vi "Write PWM.vi"(8 "Back Right":dbl, 9 "Front Right":dbl, 10 "Back Left":dbl, 11 "Front Left":dbl) -> ()   [LabVIEW 2017]
uses:
  <vilib>/myRIO/Instrument Drivers/Onboard IO/DIO/typedefs/DIO Reference.ctl
  <vilib>/myRIO/Common/Instrument Driver Framework/Utilities/typedefs/myRIO Generic Hardware Reference.ctl
  <vilib>/myRIO/Common/Instrument Driver Framework/Utilities/typedefs/Hardware Version Enum.ctl
  <vilib>/myRIO/Common/Instrument Driver Framework/Utilities/typedefs/myRIO v1.0 Reference.ctl
  <vilib>/myRIO/Common/Instrument Driver Framework/Utilities/typedefs/Generic FPGA Reference.ctl
  <vilib>/myRIO/Common/Instrument Driver Framework/myRIO v1.0/DIO/typedefs/DIO Channels List.ctl
  <vilib>/myRIO/Common/Instrument Driver Framework/myRIO v1.0/DIO/typedefs/DIO Channels Enum.ctl
  <vilib>/userdefined/High Color/nirio_resource_hc.ctl
  <vilib>/myRIO/Instrument Drivers/Onboard IO/PWM/typedefs/PWM Reference.ctl
  <vilib>/myRIO/Common/Instrument Driver Framework/myRIO v1.0/PWM/typedefs/PWM Channels Enum.ctl
  <vilib>/myRIO/Instrument Drivers/Onboard IO/PWM/typedefs/PWM Configuration.ctl
  <vilib>/myRIO/Common/Instrument Driver Framework/Utilities/vis/Is FPGA Ref Available.vi
  <vilib>/myRIO/Common/Instrument Driver Framework/myRIO v1.0/DIO/vis/myRIO v1.1 Open DIO.vi
  <vilib>/myRIO/Instrument Drivers/Onboard IO/DIO/vis/Write.vi
  <vilib>/myRIO/Common/Instrument Driver Framework/myRIO v1.0/PWM/vis/myRIO v1.1 Open PWM.vi
  <vilib>/myRIO/Instrument Drivers/Onboard IO/PWM/vis/Set Duty Cycle and Frequency.vi
  <vilib>/myRIO/Common/Instrument Driver Framework/Utilities/vis/Validate Channels.vi
  <vilib>/myRIO/Common/Instrument Driver Framework/myRIO v1.0/DIO/vis/myRIO v1.0 Reserve DIO.vi
  <vilib>/myRIO/Common/Instrument Driver Framework/myRIO v1.0/PWM/vis/myRIO v1.0 Reserve PWM.vi
  <vilib>/myRIO/Common/Instrument Driver Framework/myRIO v1.0/Resource Manager/vis/myRIO v1.0 Reserve Channel List.vi
  <vilib>/myRIO/Common/Instrument Driver Framework/myRIO v1.0/DIO/vis/myRIO v1.0 Build MUX Configuration DIO.vi
  <vilib>/myRIO/Common/Instrument Driver Framework/myRIO v1.0/PWM/vis/myRIO v1.0 Build MUX Configuration PWM.vi
  <vilib>/myRIO/Common/Instrument Driver Framework/myRIO v1.0/Resource Manager/vis/myRIO v1.0 Reserve Channel.vi
  <vilib>/myRIO/Common/Instrument Driver Framework/myRIO v1.0/Resource Manager/vis/myRIO v1.0 Unreserve Channel.vi
  <vilib>/myRIO/Common/Instrument Driver Framework/myRIO v1.0/Resource Manager/vis/myRIO v1.0 Create Configuration List.vi
  <vilib>/myRIO/Common/Instrument Driver Framework/myRIO v1.0/Resource Manager/vis/myRIO v1.0 Build Mutex Name.vi
  <vilib>/Utility/VariantDataType/GetNumericInfo.vi
  <vilib>/Utility/error.llb/Error Cluster From Error Code.vi
  <vilib>/myRIO/Common/Instrument Driver Framework/myRIO v1.0/myRIO v1.1 Open.vi
  <vilib>/myRIO/Common/Instrument Driver Framework/Utilities/vis/IO Manager.vi
  <vilib>/myRIO/Common/Instrument Driver Framework/Utilities/vis/Configuration Manager.vi
  <vilib>/myRIO/Common/Instrument Driver Framework/myRIO v1.0/Resource Manager/vis/myRIO v1.0 Configure IO.vi
  <vilib>/myRIO/Common/Instrument Driver Framework/myRIO v1.0/myRIO v1.0 Close.vi
  <vilib>/myRIO/Common/Instrument Driver Framework/myRIO v1.0/DIO/vis/myRIO v1.0 Write DIO.vi
  <vilib>/myRIO/Express VI/Onboard IO/DO/DO Express VI.xnode
  <vilib>/myRIO/Instrument Drivers/Onboard IO/DIO/vis/myRIO DIO Open.xnode
  <vilib>/myRIO/Express VI/Onboard IO/PWM/PWM Express VI.xnode
  <vilib>/myRIO/Instrument Drivers/Onboard IO/PWM/vis/myRIO PWM Open.xnode
  <vilib>/myRIO/Instrument Drivers/Onboard IO/DIO/DIO.lvlib
  <vilib>/myRIO/Instrument Drivers/Onboard IO/PWM/PWM.lvlib
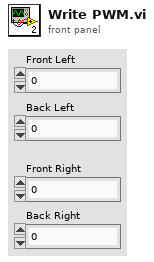
[diagram p1: front panel]
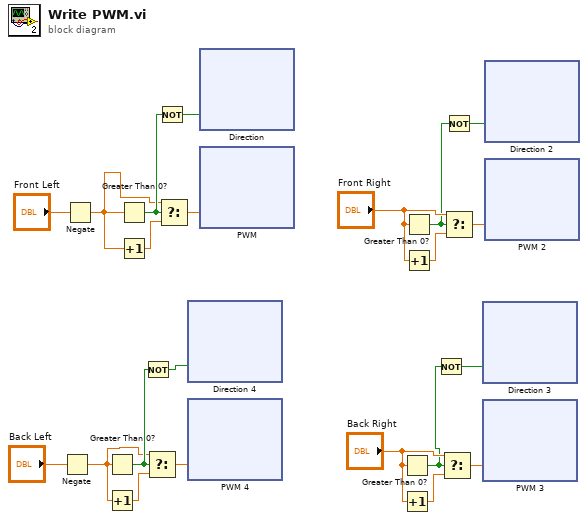
[diagram p0: block diagram]
diagram:
  n1 = Negate(x="Back Left") -> (-x=w1:dbl)
  n2 = Negate(x="Front Left") -> (-x=w4:dbl)
  n3 = Greater Than 0?(x=w1) -> (x > 0?=w7:bool)
  n4 = Increment(x=w1) -> (x+1=w19:dbl)
  n5 = Greater Than 0?(x=w4) -> (x > 0?=w11:bool)
  n6 = Increment(x=w4) -> (x+1=w22:dbl)
  n7 = Not(x=w7) -> (.not. x?=w8:bool)
  n8 = Select(t=w1, s=w7, f=w19) -> (s? t:f=w16:dbl)
  n9 = Not(x=w11) -> (.not. x?=w12:bool)
  n10 = Select(t=w4, s=w11, f=w22) -> (s? t:f=w21:dbl)
  n11 = xnode "Direction 4"("A/DIO4 (Pin 19)"=w8) -> ()  [unwired: 1 in, 1 out]
  n12 = xnode "PWM 4"("Duty Cycle"=w16) -> ()  [unwired: 1 in, 1 out]
  n13 = xnode "Direction"("B/DIO4 (Pin 19)"=w12) -> ()  [unwired: 1 in, 1 out]
  n14 = xnode "PWM"("Duty Cycle"=w21) -> ()  [unwired: 1 in, 1 out]
  n15 = Greater Than 0?(x="Back Right") -> (x > 0?=w5:bool)
  n16 = Increment(x="Back Right") -> (x+1=w20:dbl)
  n17 = Greater Than 0?(x="Front Right") -> (x > 0?=w9:bool)
  n18 = Increment(x="Front Right") -> (x+1=w18:dbl)
  n19 = Not(x=w5) -> (.not. x?=w6:bool)
  n20 = Select(t="Back Right", s=w5, f=w20) -> (s? t:f=w15:dbl)
  n21 = Not(x=w9) -> (.not. x?=w10:bool)
  n22 = Select(t="Front Right", s=w9, f=w18) -> (s? t:f=w17:dbl)
  n23 = xnode "Direction 3"("A/DIO3 (Pin 17)"=w6) -> ()  [unwired: 1 in, 1 out]
  n24 = xnode "PWM 3"("Duty Cycle"=w15) -> ()  [unwired: 1 in, 1 out]
  n25 = xnode "Direction 2"("B/DIO3 (Pin 17)"=w10) -> ()  [unwired: 1 in, 1 out]
  n26 = xnode "PWM 2"("Duty Cycle"=w17) -> ()  [unwired: 1 in, 1 out]
